vi "Email_Sender_for_Out_off_range.vi"(10 "Out of range ?":bool[](array[boolean]), 11 "Product Code/":cluster{string, "ACTUAL  PLC COUNT":i32}[](array[cluster])) -> (3 "String":string)   [LabVIEW 2017]
uses:
  4a2fb06e-711d-4851-8617-d0d2dfbe8f16.vi
  <vilib>/smtpClient/LabVIEWSMTPClient.lvlib
  <vilib>/smtpClient/Set Message Text.vi
panel:
  in  "Configure Server":bool
  in  "Enable TLS":bool
  in  "Password":string
  in  "Username":string
  in  "Port":string
  in  "Sender's Email Address":string
  in  "Outgoing Mail Server (SMTP)":string
  in  "Message":string
  in  "Subject":string
  in  "To:":string
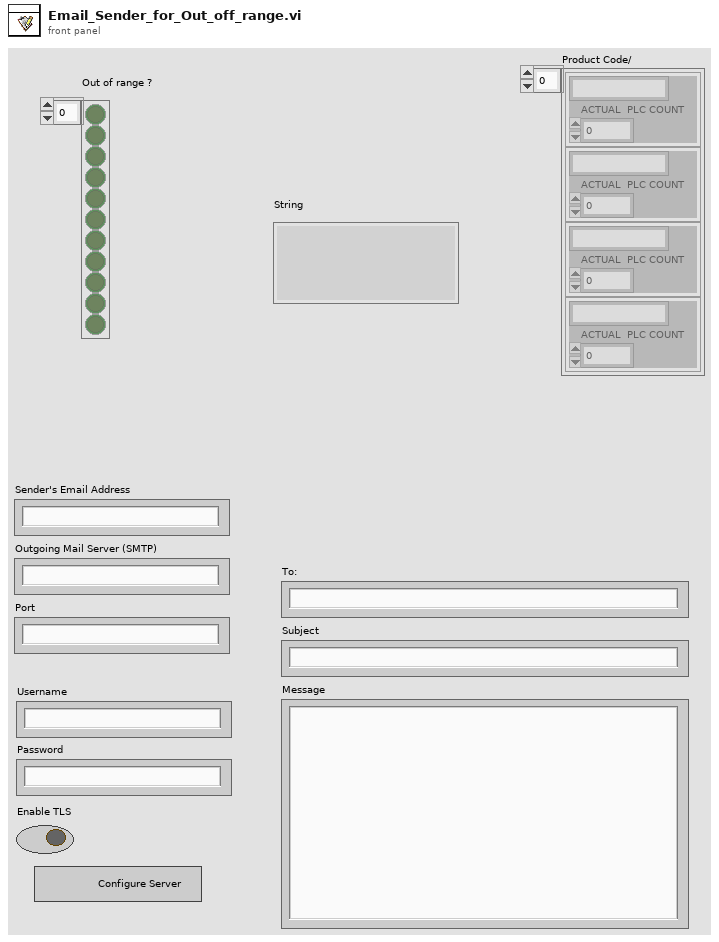
[diagram p1: front panel]
types:
  T1 = typedef "LabVIEWSMTPClient.lvlib/SmtpClientHandle.ctl" = refnum<k1>
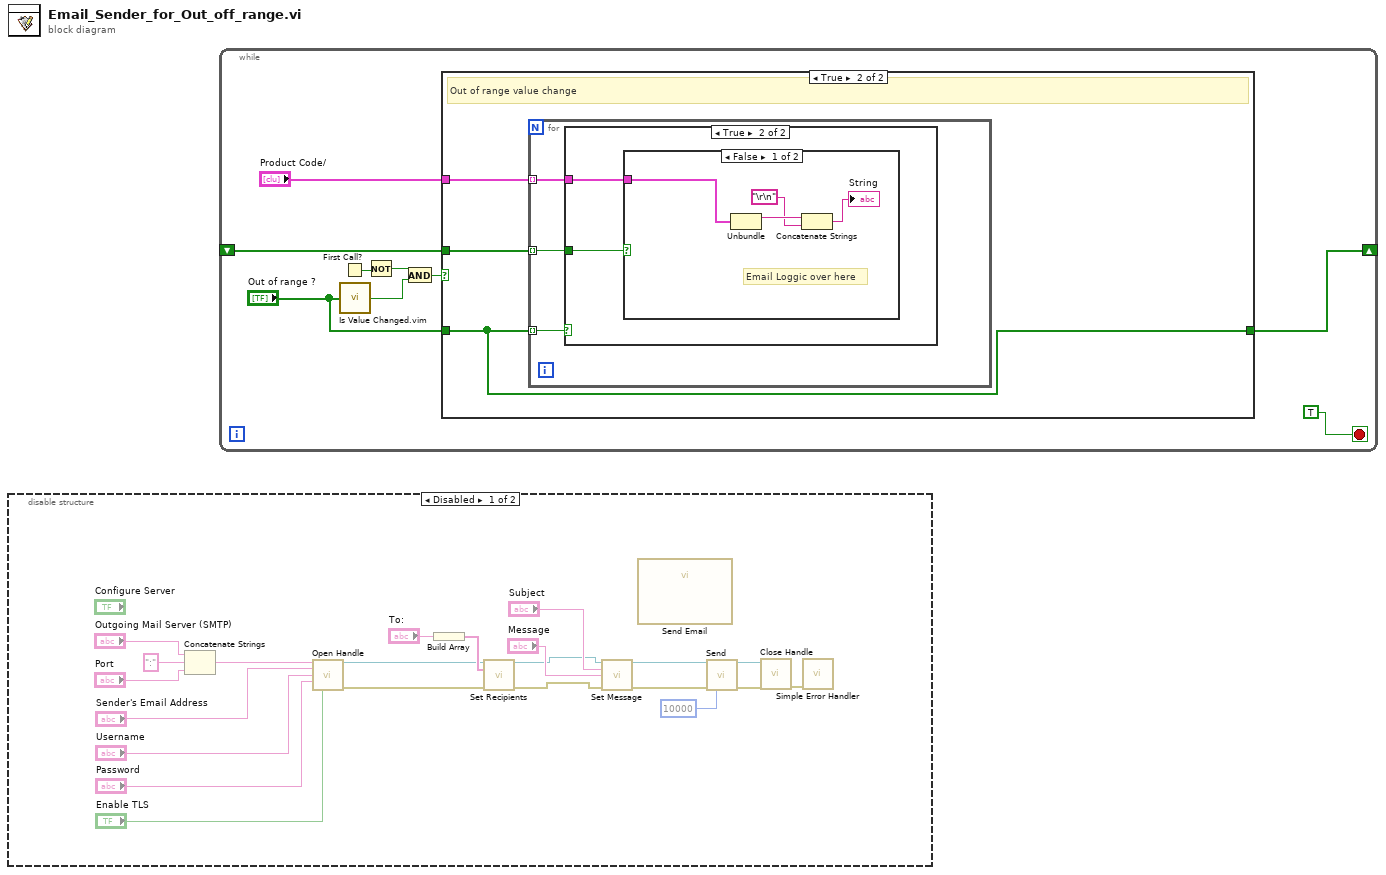
[diagram p0: block diagram]
diagram:
  n1 = disable-structure shown="Disabled" {
    frame Disabled {
      n2 = Concatenate Strings("Outgoing Mail Server (SMTP)", ":" ("string"), "Port") -> (w10:string)
      n3 = call <vilib>:"Open Handle.vi"("server address"=w10, "from"="Sender's Email Address", "username"="Username", "password"="Password", "use TLS (false)"="Enable TLS") -> ("handle out"=w3:T1, "error out"=w2:errorcluster)  [unwired: 9 in]
      n4 = Build Array("To:") -> (w20:string[])
      n5 = call <vilib>:"Set Recipients.vi"("handle in"=w3, "to"=w20, "error in (no error)"=w2) -> ("handle out"=w4:T1, "error out"=w5:errorcluster)  [unwired: 11 in]
      n6 = call-poly <vilib>:"Set Message.vi"("handle in"=w4, "subject"="Subject", "plain text message"="Message", "error in (no error)"=w5) -> ("handle out"=w16:T1, "error out"=w17:errorcluster)  [unwired: 10 in]
      n7 = call "Send Email"() -> ()  [unwired: 11 in, 1 out]
      n8 = call <vilib>:"Send.vi"("handle in"=w16, "error in (no error)"=w17, "timeout in ms (10000)"=10000 ("timeout in ms")) -> ("handle out"=w6:T1, "error out"=w1:errorcluster)  [unwired: 10 in, 1 out]
      n9 = call <vilib>:"Close Handle.vi"("handle in"=w6, "error in (no error)"=w1) -> ("error out"=w22:errorcluster)  [unwired: 12 in, 1 out]
      n10 = call <vilib>:"Simple Error Handler.vi"("error in (no error)"=w22) -> ()  [unwired: 4 in, 5 out]
    }
    frame Enabled {
    }
  }
  n11 = while {
    shift-right: [w25] -> _
    shift-left: _ -> [w24]
    stop <- TRUE stop-if-true
    n12 = First Call?() -> (First Call?: T/F=w31:bool)
    n13 = call "Is Value Changed.vim"("value"="Out of range ?") -> ("changed or first call?"=w29:bool)
    n14 = Not(x=w31) -> (.not. x?=w30:bool)
    n15 = And(x=w30, y=w29) -> (x .and. y?=w28:bool)
    n16 = case shown="True" w28 {
      tunnel: "Out of range ?" -> [w32 w34]
      tunnel: "Product Code/" -> [_ w35]
      tunnel: [w32 w34] -> w25
      tunnel: w24 -> [_ w33]
      frame False {
      }
      frame True {
        # "Out of range value change"
        n17 = for {
          tunnel: w34 -> [w37] mode=indexing
          tunnel: w35 -> [w38] mode=indexing
          tunnel: w33 -> [w36] mode=indexing
          n18 = case shown="True" w37 {
            tunnel: w38 -> [_ w40]
            tunnel: w36 -> [_ w39]
            frame False {
            }
            frame True {
              n19 = case shown="False" w39 {
                tunnel: w40 -> [w44 _]
                frame False {
                  # "Email Loggic over here"
                  n20 = Unbundle(w44) -> (w43:string)  [unwired: 1 out]
                  n21 = Concatenate Strings(w43, "\r\n") -> (→"String":string)
                }
                frame True {
                }
              }
            }
          }
        }
      }
    }
  }
